vi "Actor Core.vi"(8 "error in":errorcluster, 11 "SoftwareSetup in":refnum<class "SoftwareSetup.lvclass">) -> (0 "error out":errorcluster, 3 "Actor out":refnum<class "Actor.lvclass">)   [LabVIEW 2019, in "SoftwareSetup.lvlib" / "SoftwareSetup.lvclass"]
doc: "(<B>Filename</B>: Actor Framework.lvlib:Actor.lvclass:Actor Core.vi)\n\nReceives messages to the actor, reacts to them, and initiates any error handling that may shut the actor down.\n\nDescendant classes may override this VI to append parallel tasks for the actor to complete while it handles messages. Overrides use the Call Parent Method node."
uses:
  SoftwareSetup.lvclass
  C:/Program Files (x86)/National Instruments/LabVIEW 2019/vi.lib/ActorFramework/Actor/Actor.lvclass
  <vilib>/ActorFramework/Actor/Actor.lvclass
  User Manager.ctl
  DataBase.ctl
  Local Report.ctl
  Localization.ctl
  Preferences.ctl
  Multiple UUT Settings.ctl
  Sequence.ctl
  SoftwareSetup.lvclass/SoftwareSetup.ctl
  <vilib>/ActorFramework/Actor/Actor.lvclass/Actor.ctl
  <vilib>/ActorFramework/Message Enqueuer/Message Enqueuer.lvclass/Message Enqueuer.ctl
  59d55deb-56f5-4ab8-91ce-3d3ac24aba89.vi
  <vilib>/ActorFramework/Message Enqueuer/Init from Existing Queue.vi
  <vilib>/ActorFramework/Message Enqueuer/Enqueue.vi
  SystemSetup/SystemSetup Messages/RefreshSystemConfigurationUI Msg/RefreshSystemConfigurationUI Msg.lvclass
  C:/Program Files (x86)/National Instruments/LabVIEW 2019/vi.lib/ActorFramework/Message/Message.lvclass
  SystemSetup/SystemSetup Messages/SaveSystemConfigurationUI Msg/SaveSystemConfigurationUI Msg.lvclass
  <vilib>/ActorFramework/Message Priority Queue/Priority Enqueue.vi
  <vilib>/ActorFramework/Message Enqueuer/Message Enqueuer.lvclass
  SystemSetup/SystemSetup/SystemSetup.lvclass
  SoftwareSetup.lvlib
panel:
  in  "OK":bool
  in  "Cancel":bool
  in  "Tab Control":T1(tab)
  in  "User Manager":T2
  in  "DataBase":T3
  in  "Local Report":T4
  in  "Sequence":T5
  in  "Preferences":T6
  in  "Multiple UUT Settings":T7={"Number of Tests Sockets"=1, "Synchronization"=enum."Don't Synchronize"} {"Number of Tests Sockets" min=1 step=1}
  in  "Localization":T8
  # "User Manager File"
  # "Data Link Options"
  # "Report File"
  # "Station Info"
  # "MES Info"
  # "Number of Tests Sockets"
  # "Synchronization"
  # "Select a Language:"
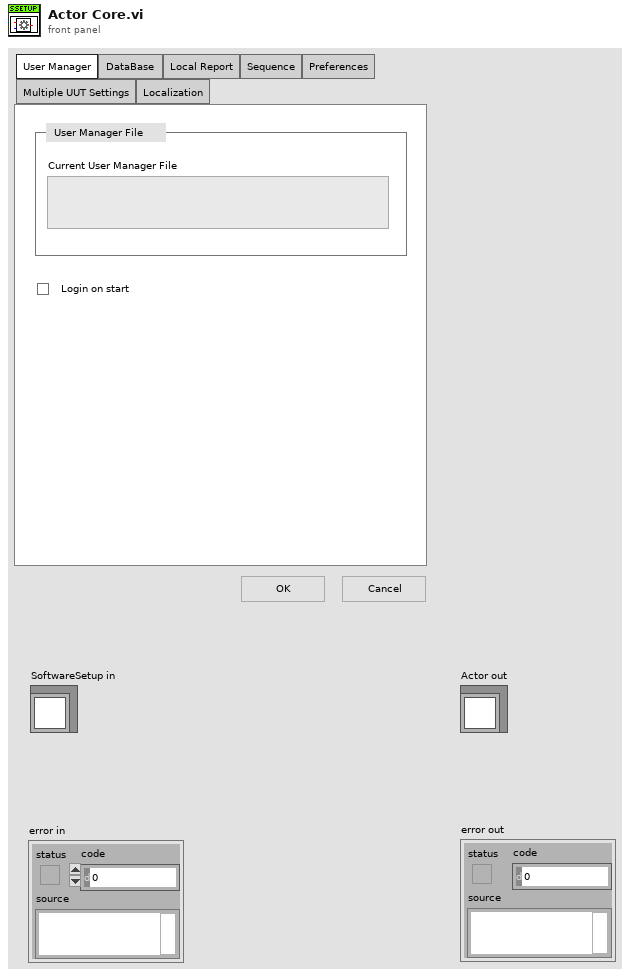
[diagram p1: front panel]
types:
  T1 = enum32{"User Manager", "DataBase ", "Local Report", "Sequence", "Preferences", "Multiple UUT Settings", "Localization"}
  T2 = typedef "SoftwareSetup.lvlib/User Manager.ctl" = cluster{"Current User Manager File":string, "Login on start":bool}
  T3 = typedef "SoftwareSetup.lvlib/DataBase.ctl" = cluster{"Connection String Expression":string, "User ID":string, "Password":string}
  T4 = typedef "SoftwareSetup.lvlib/Local Report.ctl" = cluster{"Report Path":path, "Report  Format":enum16{"CSV", "XML", "PDF", "Excel", "TXT"}, "Disabled State":bool, "Customer name":string}
  T5 = typedef "SoftwareSetup.lvlib/Sequence.ctl" = cluster{"Sequence Folder Path":path}
  T6 = typedef "SoftwareSetup.lvlib/Preferences.ctl" = cluster{"Station ID":string, "IP Address":string, "Password":string}
  T7 = typedef "SoftwareSetup.lvlib/Multiple UUT Settings.ctl" = cluster{"Number of Tests Sockets":u8, "Synchronization":enum16{"Don't Synchronize", "Serial", "Parallel", "One Thread Only"}}
  T8 = typedef "SoftwareSetup.lvlib/Localization.ctl" = cluster{"Language":enum16{"English", "Chinese"}}
  T9 = enum32{"Invalid", "Standard", "Closed", "Hidden", "Minimized", "Maximized"}
  T10 = enum32{"invalid app kind", "Development System", "Run Time System", "Student Edition", "Embedded LabVIEW", "Evaluation", "Custom"}
  T11 = cluster{"Core":cluster{"Current VI Reference":refnum<vi>, "Close Panel on Exit?":bool}, "Your Boolean data":bool, "Your string data":string}
  T12 = cluster{"Current VI Reference":refnum<vi>, "Close Panel on Exit?":bool}
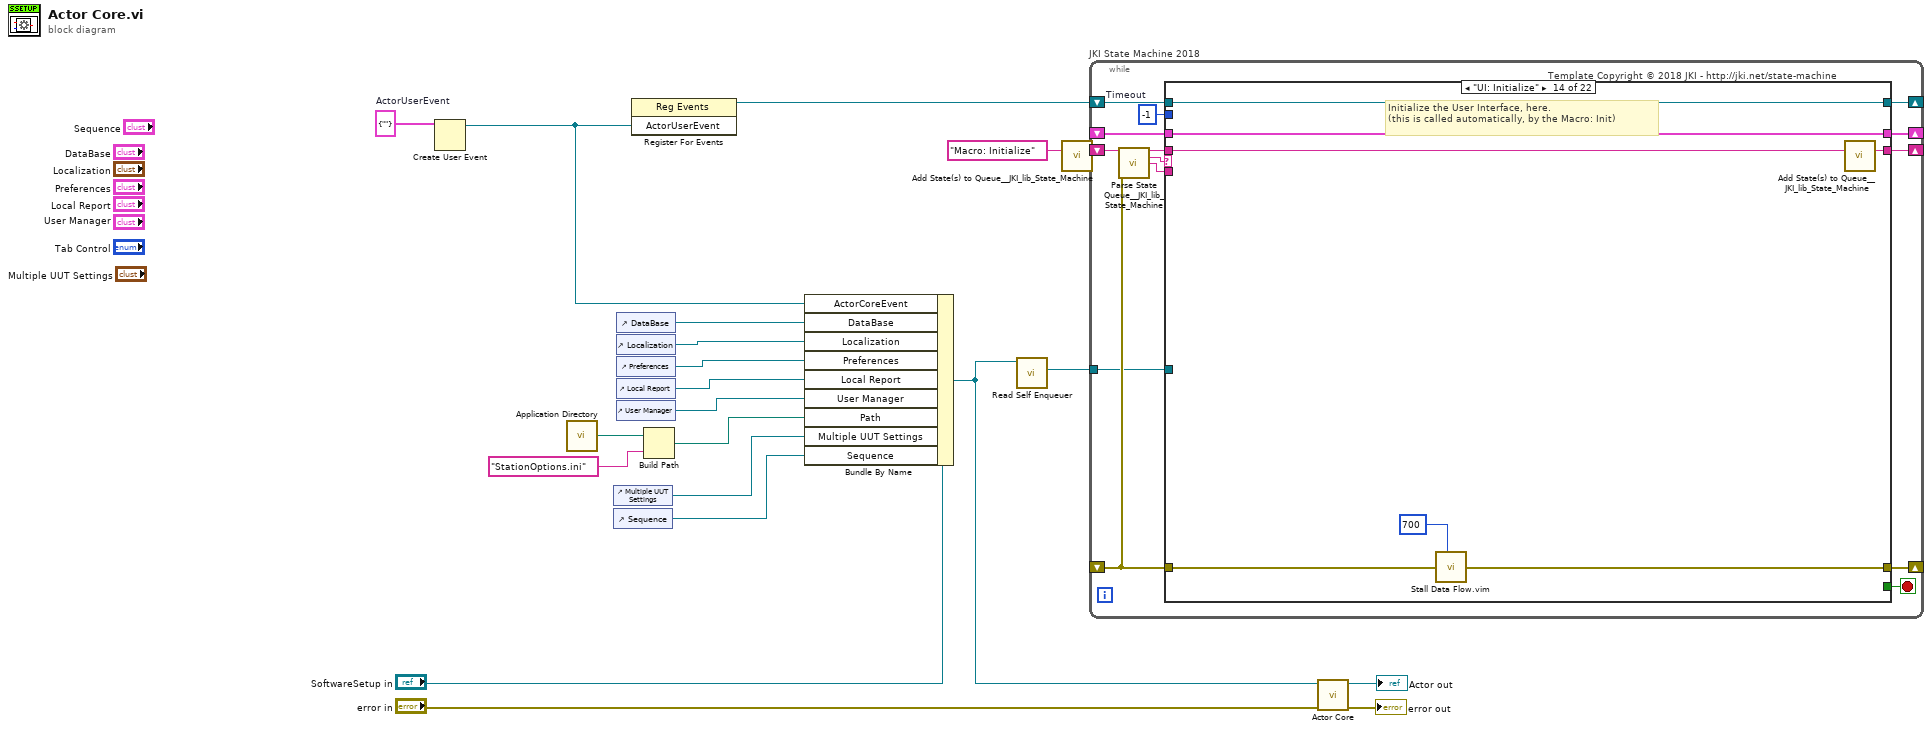
[diagram p0: block diagram]
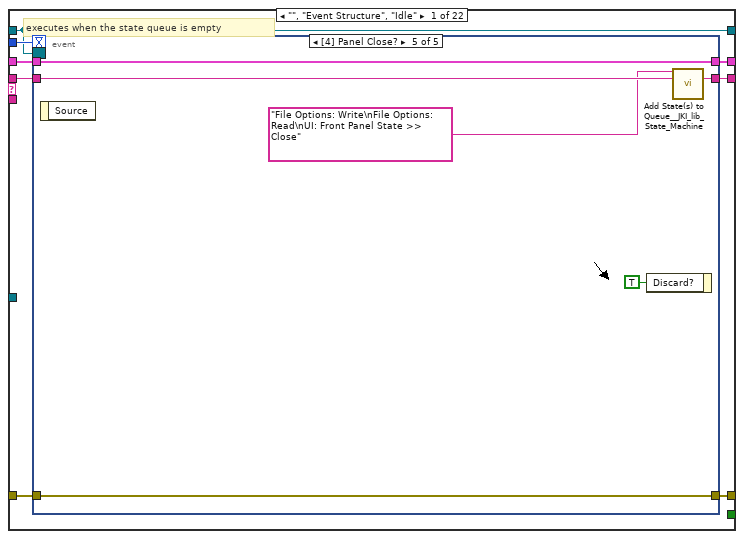
[diagram p2: hidden frame]
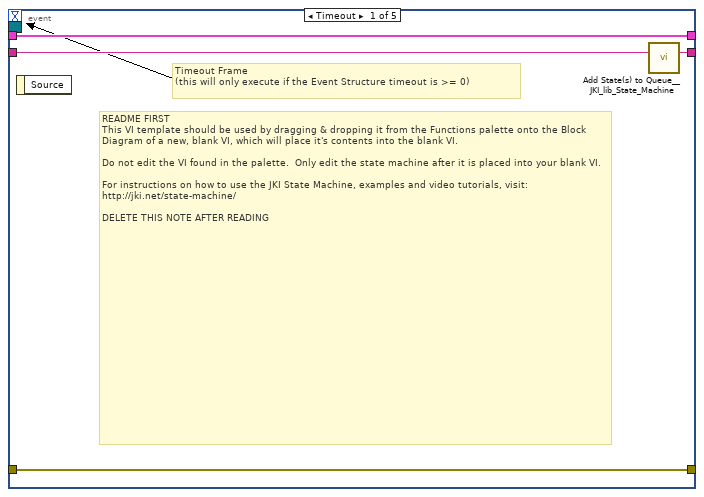
[diagram p3: hidden frame]
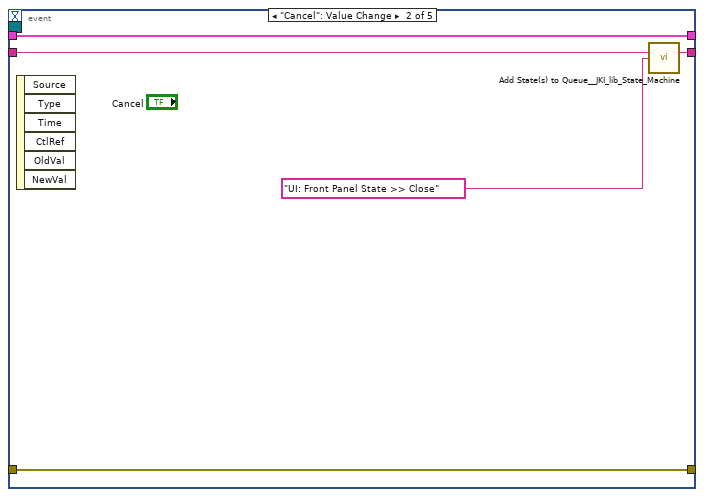
[diagram p4: hidden frame]
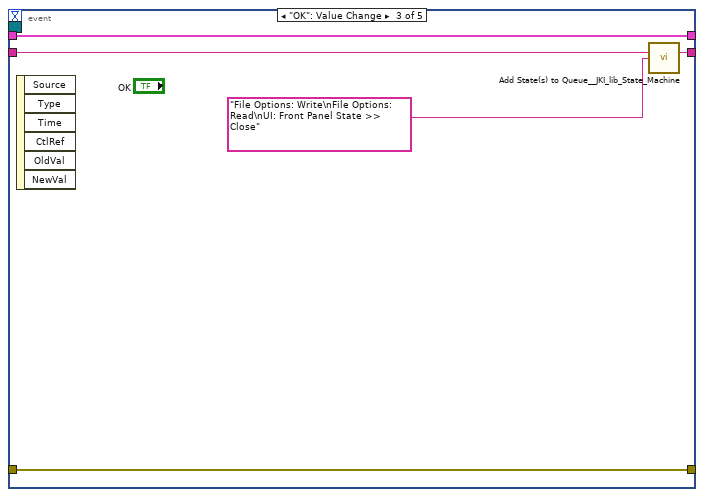
[diagram p5: hidden frame]
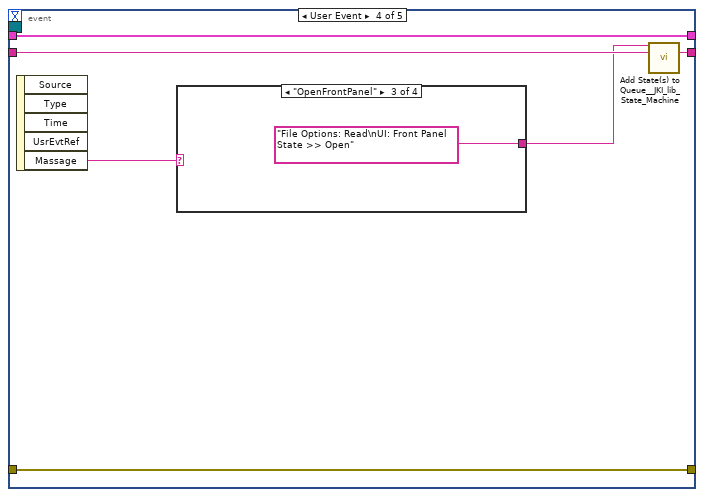
[diagram p6: hidden frame]
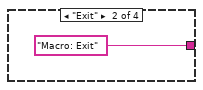
[diagram p8: hidden frame]
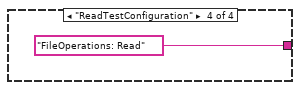
[diagram p9: hidden frame]
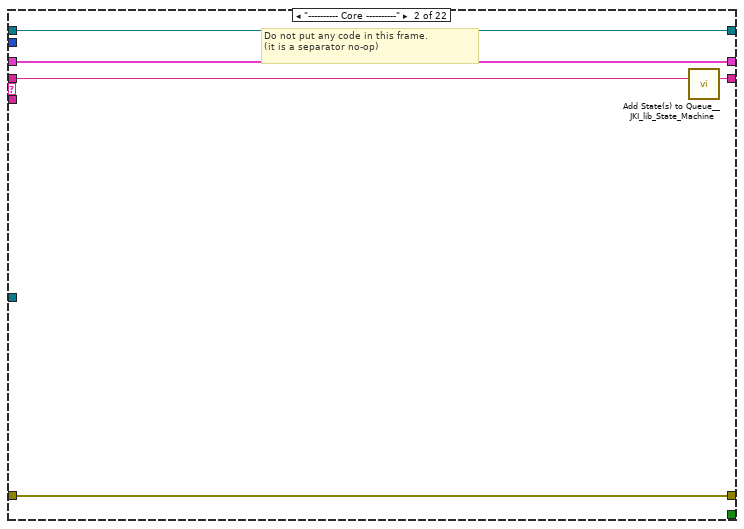
[diagram p10: hidden frame]
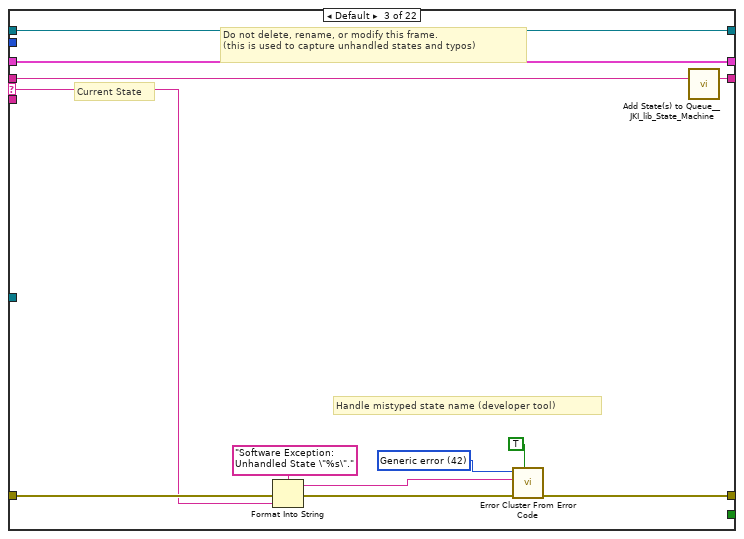
[diagram p11: hidden frame]
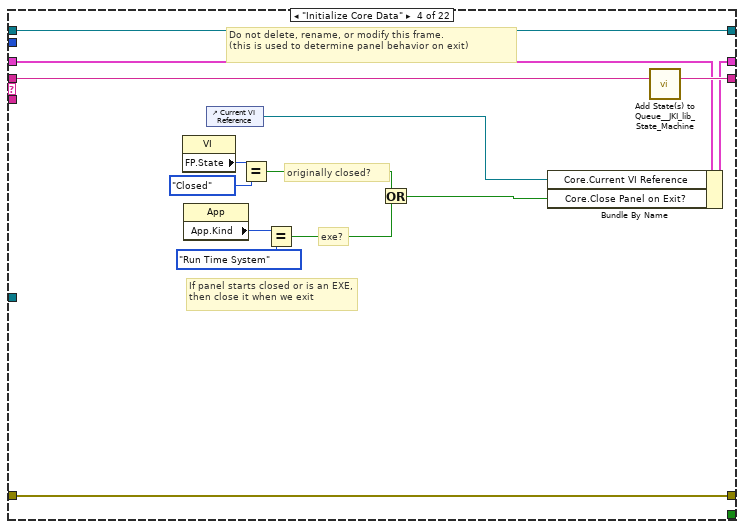
[diagram p12: hidden frame]
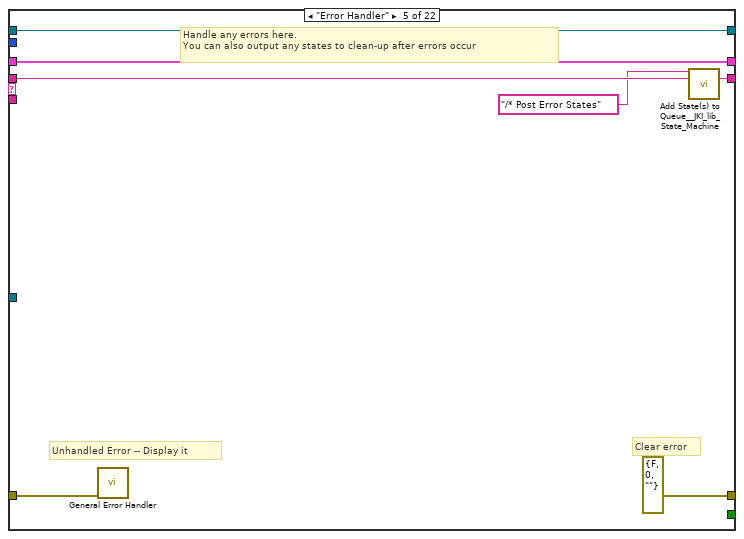
[diagram p13: hidden frame]
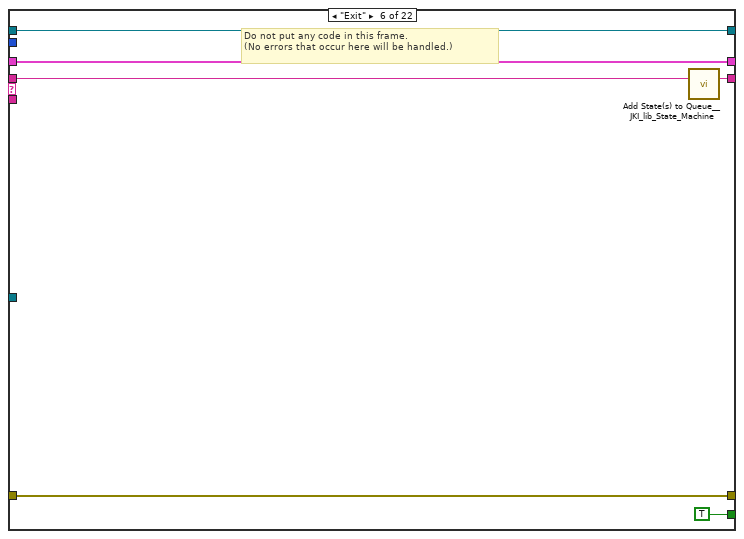
[diagram p14: hidden frame]
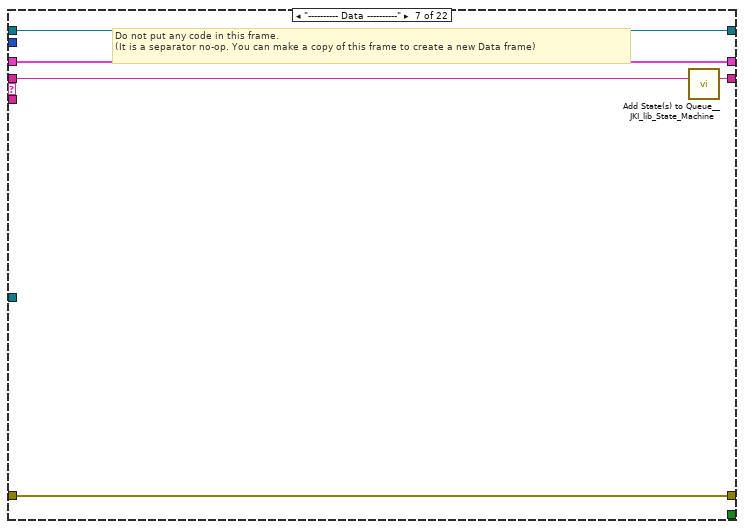
[diagram p15: hidden frame]
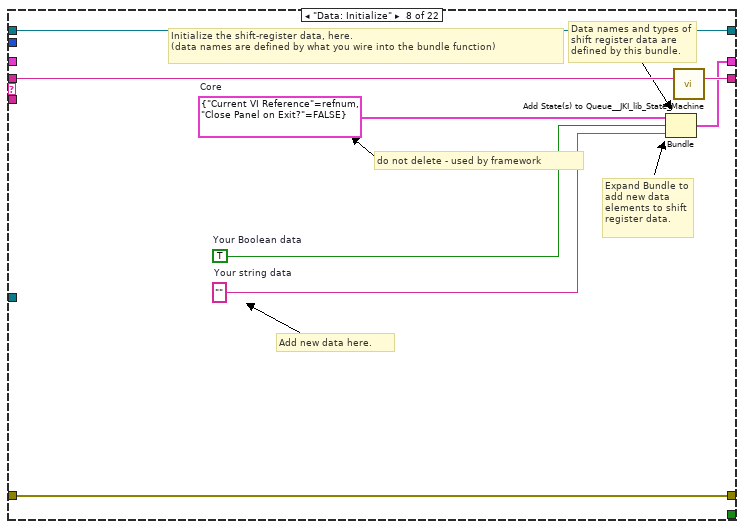
[diagram p16: hidden frame]
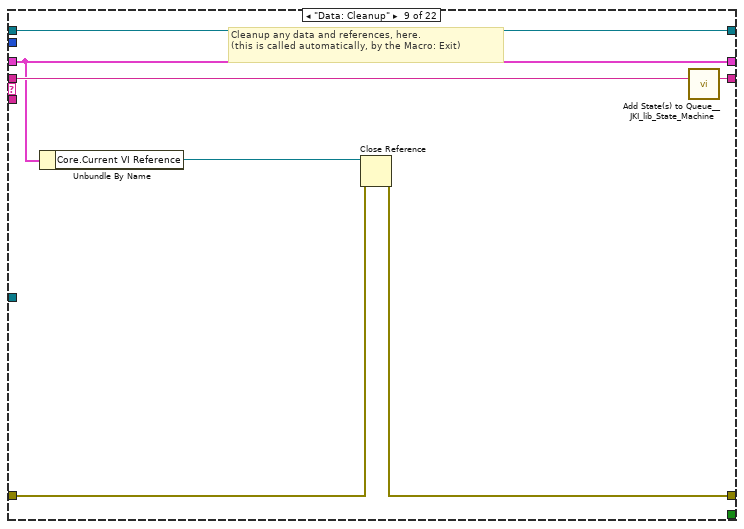
[diagram p17: hidden frame]
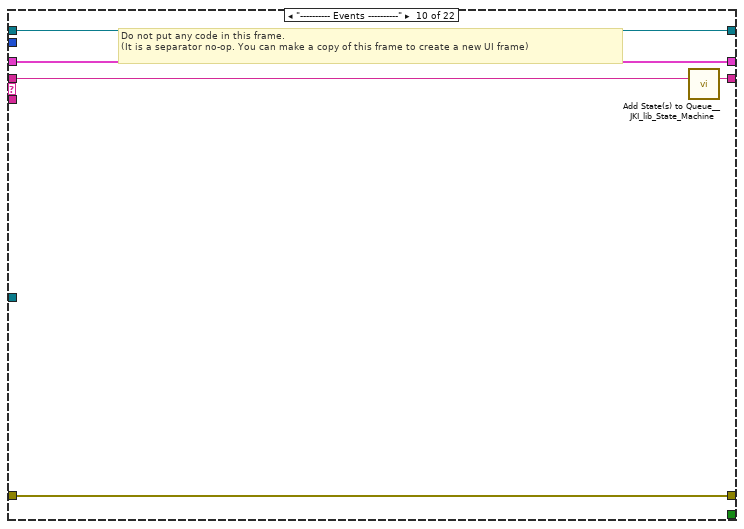
[diagram p18: hidden frame]
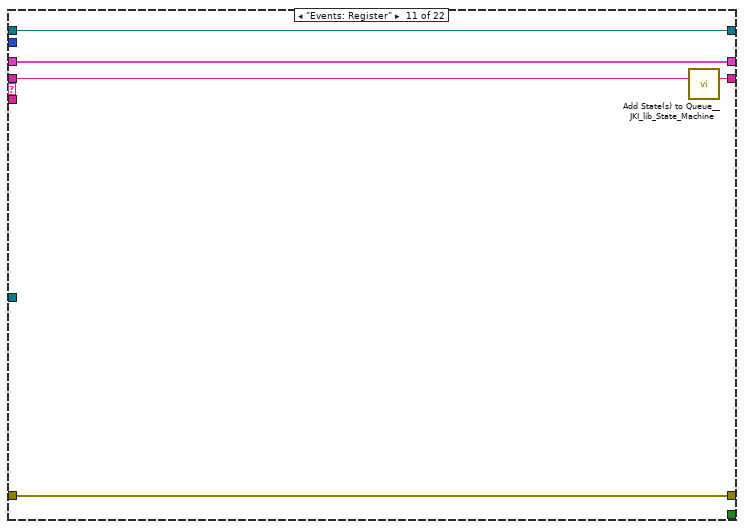
[diagram p19: hidden frame]
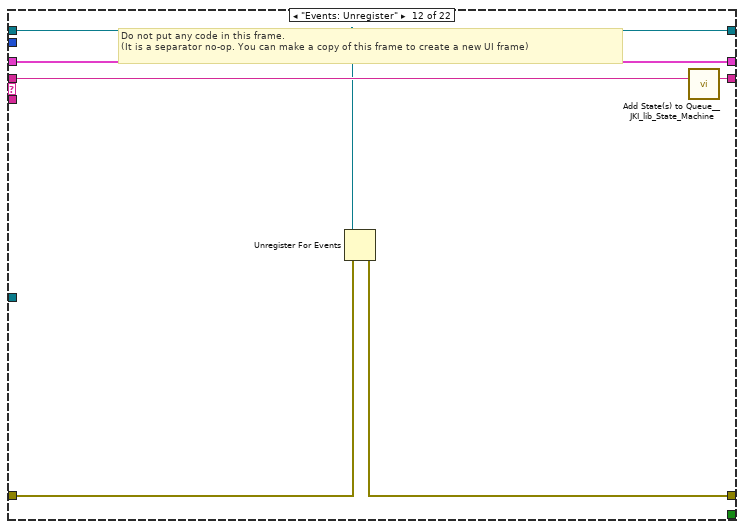
[diagram p20: hidden frame]
diagram:
  w16 = cluster{"Massage":string} {"Massage"=""}  # ActorUserEvent
  n1 = Create User Event(user event datatype=w16) -> (user event=w13:refnum<user-event>)  [unwired: 1 in, 1 out]
  n2 = call <vilib>:"Application Directory.vi"() -> ("Application Directory"=w5:path)
  n3 = control-ref of="Multiple UUT Settings"() -> (w2:refnum<vi>)
  n4 = control-ref of="Sequence"() -> (w1:refnum<vi>)
  n5 = control-ref of="DataBase"() -> (w10:refnum<vi>)
  n6 = control-ref of="Localization"() -> (w9:refnum<vi>)
  n7 = control-ref of="Preferences"() -> (w8:refnum<vi>)
  n8 = control-ref of="Local Report"() -> (w7:refnum<vi>)
  n9 = control-ref of="User Manager"() -> (w6:refnum<vi>)
  n10 = register-events(w13) -> (reference out=w15:refnum<event-registration>)  [unwired: 2 in, 1 out]
  n11 = Build Path(base path=w5, name or relative path="StationOptions.ini") -> (appended path=w4:path)
  n12 = Bundle By Name(cluster="SoftwareSetup in", "ActorCoreEvent"=w13, "DataBase"=w10, "Localization"=w9, "Preferences"=w8, "Local Report"=w7, "User Manager"=w6, "Path"=w4, "Multiple UUT Settings"=w2, "Sequence"=w1) -> (w12:refnum<class "SoftwareSetup.lvclass">)
  n13 = call <vilib>:"Read Self Enqueuer.vi"("Actor"=w12) -> ("Self Enqueuer"=w11:refnum<class "Message Enqueuer.lvclass">)  [unwired: 10 in]
  n14 = call <vilib>:"Add State(s) to Queue__JKI_lib_State_Machine.vi"("State(s) in (\"\")"="Macro: Initialize") -> ("States Out"=w18:string)  [unwired: 14 in]
  n15 = while "JKI State Machine 2018" {
    shift-right: [w28] -> _
    shift-left: _ -> [w27]
    shift-right: [w31] -> _
    shift-left: _ -> [w25]
    shift-right: [w30] -> _
    shift-left: w18 -> [w32]
    shift-right: [w24] -> _
    shift-left: w15 -> [w23]
    tunnel: w11 -> [w22]
    stop <- w29 stop-if-true
    w26 = -1  # Timeout
    # "Template Copyright © 2018 JKI - http://jki.net/state-machine"
    n16 = call <vilib>:"Parse State Queue__JKI_lib_State_Machine.vi"("State Queue"=w32, "Error In (no error)"=w25) -> ("Remaining States"=w34:string, "Current State"=w35:string, "Arguments"=w33:string)  [unwired: 11 in]
    n17 = case shown="\"UI: Initialize\"" w35 {
      selector: w35 -> [_ _ w79 _ _ _ _ _ _ _ _ _ _ _ _ _ _ _ _ _ _ _]
      tunnel: w34 -> [w43 w77 w83 w103 w110 w116 w121 w129 w136 w141 w146 w152 w157 w164 w171 w183 w253 w259 w270 w275 w281 w287]
      tunnel: w33 -> [_ _ _ _ _ _ _ _ _ _ _ _ _ _ w166 w177 _ _ _ _ _ _]
      tunnel: w27 -> [w41 w74 w81 w96 w107 w114 w118 _ w131 w138 w144 w150 w154 w162 w169 w179 w250 w256 w267 w272 w279 w284]
      tunnel: [w40 w75 w85 w100 errorcluster {"status"=FALSE, "code"=0, "source"=""} ("error out") w113 w119 w126 w132 w139 w142 w147 w155 w158 w167 w180 w251 w257 w268 w273 w276 w285] -> w31
      tunnel: w25 -> [w39 w75 w84 w100 w106 w113 w119 w126 w133 w139 w142 w148 w155 w159 w168 w181 w251 w257 w268 w273 w276 w285]
      tunnel: [w42 w76 w82 w102 w109 w115 w120 w128 w135 w140 w145 w151 w156 w163 w170 w182 w252 w258 w269 w274 w280 w286] -> w30
      tunnel: [_ _ _ _ _ TRUE _ _ _ _ _ _ _ _ _ _ _ _ _ _ _ _] -> w29
      tunnel: [w38 w74 w81 w101 w107 w114 w118 w127 w131 w138 w144 w150 w154 w162 w169 w179 w250 w256 w267 w272 w279 w284] -> w28
      tunnel: w26 -> [w37 _ _ _ _ _ _ _ _ _ _ _ _ _ _ _ _ _ _ _ _ _]
      tunnel: [w36 w73 w78 w90 w104 w111 w117 w122 w130 w137 w143 w149 w153 w161 w165 w176 w249 w254 w260 w271 w278 w283] -> w24
      tunnel: w23 -> [w36 w73 w78 w90 w104 w111 w117 w122 w130 w137 w143 w149 w153 w161 w165 w176 w249 w254 w260 w271 w278 w283]
      tunnel: w22 -> [_ _ _ _ _ _ _ _ _ _ _ _ _ _ _ _ _ _ _ _ w277 w282]
      frame "", "Event Structure", "Idle" {
        # "executes when the state queue is empty"
        n18 = event shown="[4] Panel Close?" {
          selector: w36 -> [_ _ _ _ _]
          dyn-events: _ -> [_ _ _ _ _]
          timeout: w37 -> [_ _ _ _ _]
          tunnel: w43 -> [w47 w52 w57 w63 w72]
          tunnel: [w46 w51 w56 w62 w71] -> w42
          tunnel: w41 -> [w44 w49 w54 w60 w69]
          tunnel: [w45 w50 w55 w61 w70] -> w40
          tunnel: w39 -> [w45 w50 w55 w61 w70]
          tunnel: [w44 w49 w54 w60 w69] -> w38
          event Timeout {
            # "README FIRST\nThis VI template should be used by dragging & dropping it from the Functions palette onto the Block Diagram of a new, blank VI, which will place it's contents into the blank VI.\n\nDo not edit the VI found in the palette.  Only edit the state machine after it is placed into your blank VI.\n\nFor instructions on how to use the JKI State Machine, examples and video tutorials, visit:\nhttp://jki.net/state-machine/\n\nDELETE THIS NOTE AFTER READING"
            # "Timeout Frame\n(this will only execute if the Event Structure timeout is >= 0)"
            n19 = event-data() -> ()  [unwired: 1 in, 1 out]
            n20 = call <vilib>:"Add State(s) to Queue__JKI_lib_State_Machine.vi"("State(s) in (\"\")"=w47) -> ("States Out"=w46:string)  [unwired: 14 in]
          }
          event "Cancel": Value Change {
            n21 = event-data() -> ()  [unwired: 1 in, 6 out]
            n22 = call <vilib>:"Add State(s) to Queue__JKI_lib_State_Machine.vi"("State(s) in (\"\")"=w52, "State(s) at Back (\"\")"="UI: Front Panel State >> Close") -> ("States Out"=w51:string)  [unwired: 13 in]
          }
          event "OK": Value Change {
            n23 = event-data() -> ()  [unwired: 1 in, 6 out]
            n24 = call <vilib>:"Add State(s) to Queue__JKI_lib_State_Machine.vi"("State(s) in (\"\")"=w57, "State(s) at Back (\"\")"="File Options: Write\nFile Options: Read\nUI: Front Panel State >> Close") -> ("States Out"=w56:string)  [unwired: 13 in]
          }
          event User Event {
            n25 = event-data() -> ("Massage"=w59:string)  [unwired: 1 in, 4 out]
            n26 = case shown="\"OpenFrontPanel\"" w59 {
              tunnel: [_ "Macro: Exit" "File Options: Read\nUI: Front Panel State >> Open" "FileOperations: Read"] -> w58
              frame "Idle", Default {
              }
              frame "Exit" {
              }
              frame "OpenFrontPanel" {
              }
              frame "ReadTestConfiguration" {
              }
            }
            n27 = call <vilib>:"Add State(s) to Queue__JKI_lib_State_Machine.vi"("State(s) in Front (\"\")"=w58, "State(s) in (\"\")"=w63) -> ("States Out"=w62:string)  [unwired: 13 in]
          }
          event Panel Close? {
            n28 = event-data() -> ()  [unwired: 1 in, 1 out]
            n29 = event-data("Discard?"=TRUE) -> ()  [unwired: 1 in, 1 out]
            n30 = call <vilib>:"Add State(s) to Queue__JKI_lib_State_Machine.vi"("State(s) in Front (\"\")"="File Options: Write\nFile Options: Read\nUI: Front Panel State >> Close", "State(s) in (\"\")"=w72) -> ("States Out"=w71:string)  [unwired: 13 in]
          }
        }
      }
      frame "---------- Core ----------" {
        # "Do not put any code in this frame.\n(it is a separator no-op)"
        n31 = call <vilib>:"Add State(s) to Queue__JKI_lib_State_Machine.vi"("State(s) in (\"\")"=w77) -> ("States Out"=w76:string)  [unwired: 14 in]
      }
      frame Default {
        w88 = 42 items=["No error", "Argument error", "Memory is full", "Out of zone", "End of file", "File already open", "Generic file I/O error", "File not found", "File permission error", "Disk is full", "Duplicate path", "Too many files open", "System feature not enabled", "Resource file not found", "Cannot add resource", "Resource not found", "Image not found", "Image memory error", "Pen does not exist", "Config type invalid", "Config token not found", "Config parse error", "Config memory error", "Bad external code format", "Bad external code offset", "External code not present", "Null window", "Destroy window error", "Null menu", "Print aborted", "Bad print record", "Print driver error", "Windows error during printing", "Memory error during printing", "Print dialog error", "Generic print error", "Invalid device refnum", "Device not found", "Device parameter error", "Device unit error", "Cannot open device", "Device call aborted", "Generic error", "Cancelled by user", "Object ID too low", "Object ID too high", "Object not in heap", "Unknown heap", "Unknown object (invalid DefProc)", "Unknown object (DefProc not in table)", "Message out of range", "Invalid (null) method", "Unknown message", "Manager call not supported", "Bad address", "Network operation in progress", "Network operation timed out", "Connection is busy", "Network attribute not supported", "Network error", "Address in use", "System out of memory", "Connection aborted", "Connection refused", "Not connected", "Already connected", "Connection closed", "Initialization error (interapplication manager)", "Bad occurrence", "Wait on unbound occurrence handler", "Occurrence queue overflow", "Datalog type conflict", "Unused", "Unrecognized type (interapplication manager)", "Memory corrupt", "Failed to make temporary DLL", "Old CIN version", "Drag socket not found", "Failed to load drop-object", "Failed to register OLE object", "Failed to release OLE object", "Format specifier type mismatch", "Unknown format specifier", "Too few format specifiers", "Too many format specifiers", "Scan failed", "Newer CIN version", "Error converting to variant", "Runtime menu error", "Password tampered", "Variant attribute not found", "Incompatible variant data type", "Event data is not available", "Event Store is not present", "Occurrence is not found", "Event Queue is not created", "Event info is not available", "Refnum passed is NULL", "Error retrieving Class GUID", "Error retrieving CoClass GUID", "Error retrieving TypeLib GUID.", "Bad built application magic bytes.", "Specific driver is different from the specific driver associated with the Logical Name.", "There is no session opened to the class driver.", "Max Error", "MAX - Error with config objects", "MAX - Error loading configuration", "MAX - Group not supported"]
        # "Current State"
        # "Do not delete, rename, or modify this frame.\n(this is used to capture unhandled states and typos)"
        # "Handle mistyped state name (developer tool)"
        n32 = Format Into String(format string="Software Exception: Unhandled State \"%s\"." ("message"), error in=w84, w79) -> (resulting string=w87:string, error out=w86:errorcluster)  [unwired: 1 in]
        n33 = call <vilib>:"Error Cluster From Error Code.vi"("show call chain? (False)"=TRUE, "error in (no error)"=w86, "error message (\"\")"=w87, "error code (0)"=w88) -> ("error out"=w85:errorcluster)  [unwired: 5 in]
        n34 = call <vilib>:"Add State(s) to Queue__JKI_lib_State_Machine.vi"("State(s) in (\"\")"=w83) -> ("States Out"=w82:string)  [unwired: 14 in]
      }
      frame "Initialize Core Data" {
        # "Do not delete, rename, or modify this frame.\n(this is used to determine panel behavior on exit)"
        # "originally closed?"
        # "exe?"
        # "If panel starts closed or is an EXE, then close it when we exit"
        n35 = property class="VI"() -> ("FP.State"=w93:T9)  [unwired: 2 in, 2 out]
        n36 = property class="App"() -> ("App.Kind"=w99:T10)  [unwired: 2 in, 2 out]
        n37 = control-ref of="Current VI Reference"() -> (w94:refnum<vi>)
        n38 = Equal?(x=w93, y=T9."Closed" ("Front Panel Window:State")) -> (x = y?=w91:bool)
        n39 = Equal?(x=w99, y=T10."Run Time System" ("Application:Kind")) -> (x = y?=w97:bool)
        n40 = Or(x=w91, y=w97) -> (x .or. y?=w95:bool)
        n41 = Bundle By Name(cluster=w96, "Core.Current VI Reference"=w94, "Core.Close Panel on Exit?"=w95) -> (w101:T11)
        n42 = call <vilib>:"Add State(s) to Queue__JKI_lib_State_Machine.vi"("State(s) in (\"\")"=w103) -> ("States Out"=w102:string)  [unwired: 14 in]
      }
      frame "Error Handler" {
        # "Unhandled Error -- Display it"
        # "Handle any errors here.\nYou can also output any states to clean-up after errors occur"
        # "Clear error"
        n43 = call <vilib>:"General Error Handler.vi"("error in (no error)"=w106) -> ()  [unwired: 10 in, 5 out]
        n44 = call <vilib>:"Add State(s) to Queue__JKI_lib_State_Machine.vi"("State(s) in Front (\"\")"="/* Post Error States", "State(s) in (\"\")"=w110) -> ("States Out"=w109:string)  [unwired: 13 in]
      }
      frame "Exit" {
        # "Do not put any code in this frame.\n(No errors that occur here will be handled.)"
        n45 = call <vilib>:"Add State(s) to Queue__JKI_lib_State_Machine.vi"("State(s) in (\"\")"=w116) -> ("States Out"=w115:string)  [unwired: 14 in]
      }
      frame "---------- Data ----------" {
        # "Do not put any code in this frame.\n(It is a separator no-op. You can make a copy of this frame to create a new Data frame)"
        n46 = call <vilib>:"Add State(s) to Queue__JKI_lib_State_Machine.vi"("State(s) in (\"\")"=w121) -> ("States Out"=w120:string)  [unwired: 14 in]
      }
      frame "Data: Initialize" {
        w123 = T12 {"Current VI Reference"=refnum, "Close Panel on Exit?"=FALSE}  # Core
        w125 = TRUE  # Your Boolean data
        w124 = ""  # Your string data
        # "do not delete - used by framework"
        # "Expand Bundle to add new data elements to shift register data."
        # "Add new data here."
        # "Data names and types of shift register data are defined by this bundle."
        # "Initialize the shift-register data, here.\n(data names are defined by what you wire into the bundle function)"
        n47 = Bundle("Core"=w123, "Your Boolean data"=w125, "Your string data"=w124) -> (w127:T11)  [unwired: 1 in]
        n48 = call <vilib>:"Add State(s) to Queue__JKI_lib_State_Machine.vi"("State(s) in (\"\")"=w129) -> ("States Out"=w128:string)  [unwired: 14 in]
      }
      frame "Data: Cleanup" {
        # "Cleanup any data and references, here.\n(this is called automatically, by the Macro: Exit)"
        n49 = Unbundle By Name(w131) -> ("Core.Current VI Reference"=w134:refnum<vi>)
        n50 = Close Reference(reference=w134, error in (no error)=w133) -> (error out=w132:errorcluster)
        n51 = call <vilib>:"Add State(s) to Queue__JKI_lib_State_Machine.vi"("State(s) in (\"\")"=w136) -> ("States Out"=w135:string)  [unwired: 14 in]
      }
      frame "---------- Events ----------" {
        # "Do not put any code in this frame.\n(It is a separator no-op. You can make a copy of this frame to create a new UI frame)"
        n52 = call <vilib>:"Add State(s) to Queue__JKI_lib_State_Machine.vi"("State(s) in (\"\")"=w141) -> ("States Out"=w140:string)  [unwired: 14 in]
      }
      frame "Events: Register" {
        n53 = call <vilib>:"Add State(s) to Queue__JKI_lib_State_Machine.vi"("State(s) in (\"\")"=w146) -> ("States Out"=w145:string)  [unwired: 14 in]
      }
      frame "Events: Unregister" {
        # "Do not put any code in this frame.\n(It is a separator no-op. You can make a copy of this frame to create a new UI frame)"
        n54 = Unregister For Events(event registration refnum=w149, error in=w148) -> (error out=w147:errorcluster)
        n55 = call <vilib>:"Add State(s) to Queue__JKI_lib_State_Machine.vi"("State(s) in (\"\")"=w152) -> ("States Out"=w151:string)  [unwired: 14 in]
      }
      frame "---------- UI ----------" {
        # "Do not put any code in this frame.\n(It is a separator no-op. You can make a copy of this frame to create a new UI frame)"
        n56 = call <vilib>:"Add State(s) to Queue__JKI_lib_State_Machine.vi"("State(s) in (\"\")"=w157) -> ("States Out"=w156:string)  [unwired: 14 in]
      }
      frame "UI: Initialize" {
        # "Initialize the User Interface, here.\n(this is called automatically, by the Macro: Init)"
        n57 = call "Stall Data Flow.vim"("value in"=w159, "milliseconds to wait"=u32 700) -> ("value out"=w158:errorcluster)  [unwired: 1 out]
        n58 = call <vilib>:"Add State(s) to Queue__JKI_lib_State_Machine.vi"("State(s) in (\"\")"=w164) -> ("States Out"=w163:string)  [unwired: 14 in]
      }
      frame "UI: Cursor Set" {
        # "Argument"
        # "Set and Unset Cursor Busy.\n(Usage: \"UI: Cursor Set >> Busy|Idle\")"
        n59 = case shown="\"Idle\", Default" w166 {
          tunnel: w168 -> [w173 w175]
          tunnel: [w172 w174] -> w167
          frame "Idle", Default {
            n60 = call <vilib>:"Unset Busy.vi"("error in (no error)"=w173) -> ("error out"=w172:errorcluster)  [unwired: 10 in]
          }
          frame "Busy" {
            n61 = call <vilib>:"Set Busy.vi"("error in (no error)"=w175) -> ("error out"=w174:errorcluster)  [unwired: 9 in, 1 out]
          }
        }
        n62 = call <vilib>:"Add State(s) to Queue__JKI_lib_State_Machine.vi"("State(s) in (\"\")"=w171) -> ("States Out"=w170:string)  [unwired: 14 in]
      }
      frame "UI: Front Panel State" {
        # "Argument"
        # "Set Front Panel Open or Closed\n(Usage: \"UI: Front Panel State >> Open|Close\")"
        n63 = Unbundle By Name(w179) -> ("Core.Current VI Reference"=w178:refnum<vi>)
        n64 = case shown="\"Hidden\", \"Hide\"" w177 {
          tunnel: w181 -> [w189 w204 w215 w228 w241]
          tunnel: [w191 w205 w217 w230 w243] -> w180
          tunnel: w178 -> [w190 w202 w216 w229 w242]
          frame "Open", "Standard", Default {
            w184 = T9."Standard" ("State")
            n65 = property class="VI"(reference=w190, error in=w189) -> (reference out=w187:refnum<vi>, error out=w188:errorcluster, "FP.State"=w186:T9)
            n66 = Not Equal?(x=w186, y=w184) -> (x != y?=w185:bool)
            n67 = case shown="True" w185 {
              tunnel: [w195 w197] -> w191
              tunnel: w188 -> [w194 w197]
              tunnel: w187 -> [w193 _]
              tunnel: w184 -> [w192 _]
              frame True {
                n68 = invoke class="VI" method="FP.Open"(reference=w193, error in=w194, "Activate"=TRUE, "State"=w192) -> (error out=w195:errorcluster)  [unwired: 1 in, 4 out]
              }
              frame False {
              }
            }
          }
          frame "Close", "Closed" {
            n69 = property class="VI"(reference=w202, error in=w204) -> (reference out=w201:refnum<vi>, error out=w203:errorcluster, "FP.State"=w199:T9)
            n70 = Not Equal?(x=w199, y=T9."Closed" ("Front Panel Window:State")) -> (x != y?=w198:bool)
            n71 = case shown="True" w198 {
              tunnel: [w206 w209] -> w205
              tunnel: w203 -> [w206 w208]
              tunnel: w201 -> [_ w207]
              frame False {
              }
              frame True {
                n72 = invoke class="VI" method="FP.Close"(reference=w207, error in=w208) -> (error out=w209:errorcluster)  [unwired: 1 in, 2 out]
              }
            }
          }
          frame "Hidden", "Hide" {
            w210 = T9."Hidden" ("State")
            n73 = property class="VI"(reference=w216, error in=w215) -> (reference out=w213:refnum<vi>, error out=w214:errorcluster, "FP.State"=w212:T9)
            n74 = Not Equal?(x=w212, y=w210) -> (x != y?=w211:bool)
            n75 = case shown="True" w211 {
              tunnel: [w221 w222] -> w217
              tunnel: w214 -> [w220 w222]
              tunnel: w213 -> [w219 _]
              tunnel: w210 -> [w218 _]
              frame True {
                n76 = invoke class="VI" method="FP.Open"(reference=w219, error in=w220, "State"=w218) -> (error out=w221:errorcluster)  [unwired: 2 in, 4 out]
              }
              frame False {
              }
            }
          }
          frame "Minimize", "Minimized" {
            w223 = T9."Minimized" ("State")
            n77 = property class="VI"(reference=w229, error in=w228) -> (reference out=w226:refnum<vi>, error out=w227:errorcluster, "FP.State"=w225:T9)
            n78 = Not Equal?(x=w225, y=w223) -> (x != y?=w224:bool)
            n79 = case shown="True" w224 {
              tunnel: [w234 w235] -> w230
              tunnel: w227 -> [w233 w235]
              tunnel: w226 -> [w232 _]
              tunnel: w223 -> [w231 _]
              frame True {
                n80 = invoke class="VI" method="FP.Open"(reference=w232, error in=w233, "State"=w231) -> (error out=w234:errorcluster)  [unwired: 2 in, 4 out]
              }
              frame False {
              }
            }
          }
          frame "Maximize", "Maximized" {
            w236 = T9."Maximized" ("State")
            n81 = property class="VI"(reference=w242, error in=w241) -> (reference out=w239:refnum<vi>, error out=w240:errorcluster, "FP.State"=w238:T9)
            n82 = Not Equal?(x=w238, y=w236) -> (x != y?=w237:bool)
            n83 = case shown="True" w237 {
              tunnel: [w247 w248] -> w243
              tunnel: w240 -> [w246 w248]
              tunnel: w239 -> [w245 _]
              tunnel: w236 -> [w244 _]
              frame True {
                n84 = invoke class="VI" method="FP.Open"(reference=w245, error in=w246, "State"=w244) -> (error out=w247:errorcluster)  [unwired: 2 in, 4 out]
              }
              frame False {
              }
            }
          }
        }
        n85 = call <vilib>:"Add State(s) to Queue__JKI_lib_State_Machine.vi"("State(s) in (\"\")"=w183) -> ("States Out"=w182:string)  [unwired: 14 in]
      }
      frame "---------- Macro ----------" {
        # "Do not put any code in this frame.\n(It is a separator no-op. You can make a copy of this frame to create a new Macro frame)"
        n86 = call <vilib>:"Add State(s) to Queue__JKI_lib_State_Machine.vi"("State(s) in (\"\")"=w253) -> ("States Out"=w252:string)  [unwired: 14 in]
      }
      frame "Macro: Initialize" {
        # "Initialization Macro\n(This is called once, when the VI starts)"
        n87 = call <vilib>:"Add State(s) to Queue__JKI_lib_State_Machine.vi"("State(s) in Front (\"\")"="Data: Initialize\nInitialize Core Data\nEvents: Register\nUI: Initialize\nUI: Front Panel State >> Close\nFile Options: Read", "State(s) in (\"\")"=w259) -> ("States Out"=w258:string)  [unwired: 13 in]
      }
      frame "Macro: Exit" {
        # "Exit Macro\n(This is called once, when the VI exits)"
        n88 = Unbundle By Name(w267) -> ("Core.Close Panel on Exit?"=w266:bool)
        n89 = Select(t="UI: Front Panel State >> Close", s=w266, f="") -> (s? t:f=w263:string)
        n90 = call <vilib>:"Add State(s) to Queue__JKI_lib_State_Machine.vi"("State(s) in (\"\")"=w263, "State(s) at Back (\"\")"="Data: Cleanup\nEvents: Unregister\nExit") -> ("States Out"=w261:string)  [unwired: 13 in]
        n91 = call <vilib>:"Add State(s) to Queue__JKI_lib_State_Machine.vi"("State(s) in Front (\"\")"=w261, "State(s) in (\"\")"=w270) -> ("States Out"=w269:string)  [unwired: 13 in]
      }
      frame "---------- File Options ----------" {
        # "Template Separator\n(You can make a copy of, or modify, this frame)"
        n92 = call <vilib>:"Add State(s) to Queue__JKI_lib_State_Machine.vi"("State(s) in (\"\")"=w275) -> ("States Out"=w274:string)  [unwired: 14 in]
      }
      frame "File Options: Read" {
        # "Your code here.\n(You can make a copy of, or modify, this frame)"
        n93 = call "Send RefreshSystemConfigurationUI.vi"("error in (no error)"=w276, "Message Enqueuer"=w277) -> ()  [unwired: 8 in, 2 out]
        n94 = call <vilib>:"Add State(s) to Queue__JKI_lib_State_Machine.vi"("State(s) in (\"\")"=w281) -> ("States Out"=w280:string)  [unwired: 14 in]
      }
      frame "File Options: Write" {
        # "Your code here.\n(You can make a copy of, or modify, this frame)"
        n95 = call "Send SaveSystemConfigurationUI.vi"("Message Enqueuer"=w282) -> ()  [unwired: 9 in, 2 out]
        n96 = call <vilib>:"Add State(s) to Queue__JKI_lib_State_Machine.vi"("State(s) in (\"\")"=w287) -> ("States Out"=w286:string)  [unwired: 14 in]
      }
    }
  }
  n97 = call-parent "Actor Core.vi"("error in"="error in", "Actor in"=w12) -> ("error out"=→"error out":errorcluster, "Actor out"=→"Actor out":refnum<class "Actor.lvclass">)  [unwired: 8 in]
